vi "Actor Destroy Core.vi"(7 "Actor":refnum<class "Actor.lvclass">, 11 "Msging Self Actor State in":refnum<class "Msging Self Actor State.lvclass">) -> (0 "error out":errorcluster)   [LabVIEW 2021, in "jettl.lvlib" / "Msging Self Actor State.lvclass"]
uses:
  Msging Self Actor State.lvclass
  Actor/Actor.lvclass
  Msgs/Actor Destroy/Actor Destroy Msg Strategy/Actor Destroy Msg Strategy.lvclass
  C:/git/jettl/src/LVCAM/LVCAM/Msg Strategy/Msg Strategy.lvclass
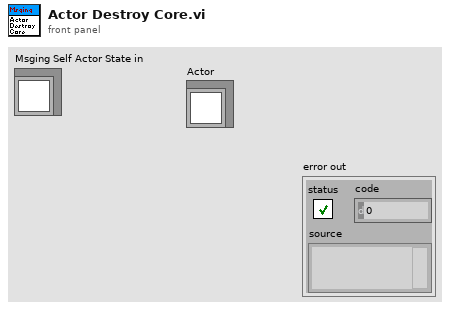
[diagram p1: front panel]
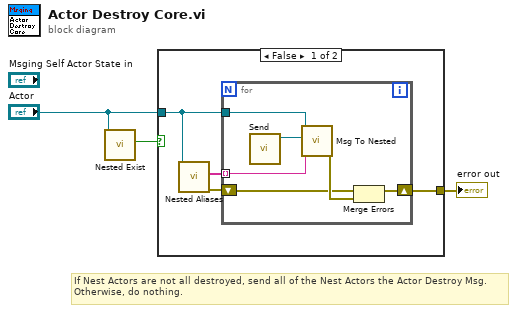
[diagram p0: block diagram]
diagram:
  # "If Nest Actors are not all destroyed, send all of the Nest Actors the Actor Destroy Msg. Otherwise, do nothing."
  n1 = call-dynamic "Nested Exist.vi"("Actor in"="Actor") -> ("Nested Exist?"=w2:bool)  [unwired: 10 in]
  n2 = case shown="False" w2 {
    tunnel: [w7 _] -> w3
    tunnel: "Actor" -> [w4 _]
    frame False {
      n3 = call-dynamic "Nested Aliases.vi"("Actor in"=w4) -> ("error out"=w5:errorcluster, "Nested Aliases"=w6:string[])  [unwired: 9 in]
      n4 = for {
        tunnel: w6 -> [w10] mode=indexing
        shift-right: [w13] -> w7
        shift-left: w5 -> [w8]
        tunnel: w4 -> [w12]
        n5 = call "Send.vi"() -> ("Actor Destroy Msg Strategy out"=w11:refnum<class "Actor Destroy Msg Strategy.lvclass">)  [unwired: 11 in]
        n6 = call-dynamic "Msg To Nested.vi"("Alias"=w10, "Msg"=w11, "Actor in"=w12) -> ("error out"=w9:errorcluster)  [unwired: 8 in]
        n7 = Merge Errors(w8, w9) -> (w13:errorcluster)
      }
    }
    frame True {
      # "there exist no Nest Actors to be destroyed, do nothing"
    }
  }
  "error out" <- w3
